vi "Read PL (2D) txt File.vi"(1 "Path":path) -> (0 "Intensity Graph":dbl[][](graph))   [LabVIEW 2011]
uses:
  <vilib>/Utility/file.llb/Read From Spreadsheet File (DBL).vi
panel:
  in  "Array":u32[](array[colorbox])
  in  "multiplier":dbl=13.79
  in  "start":dbl=13.79
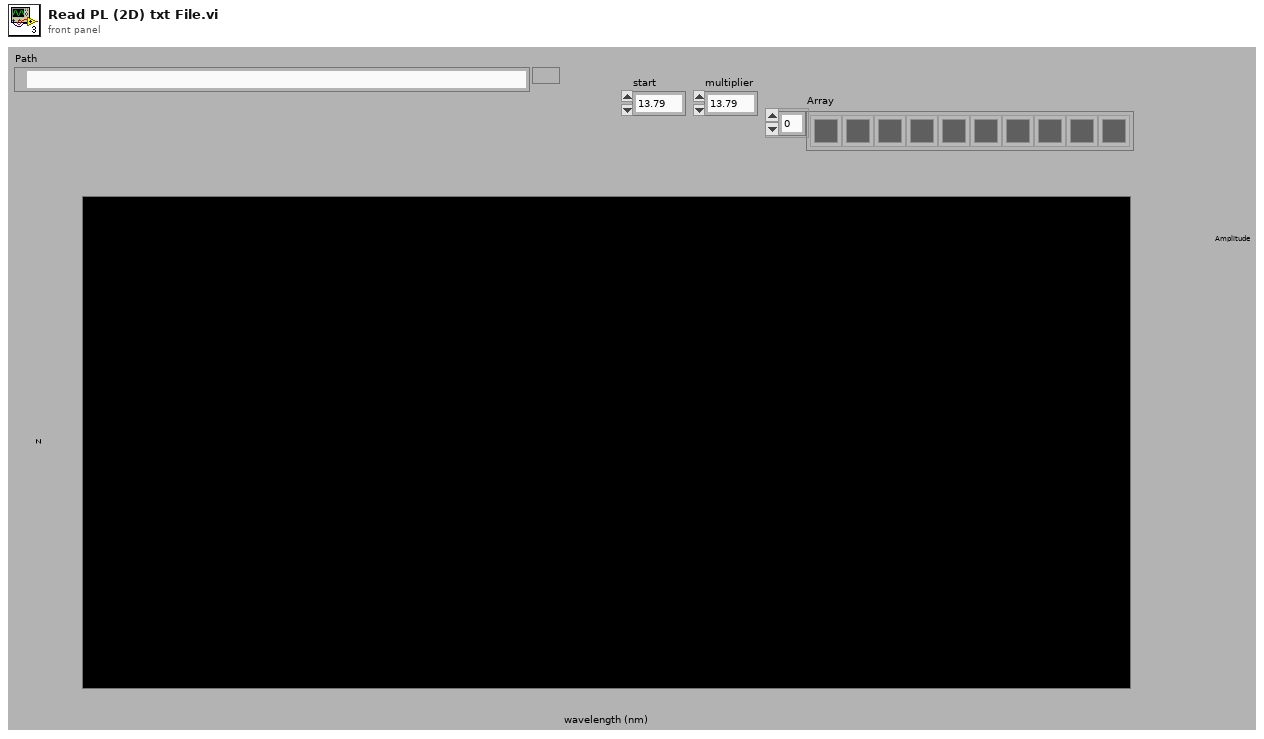
[diagram p1: front panel]
types:
  T1 = typedef "LVOffsetAndMultiplierTypeDef.ctl" = cluster{"Offset":dbl, "Multiplier":dbl}
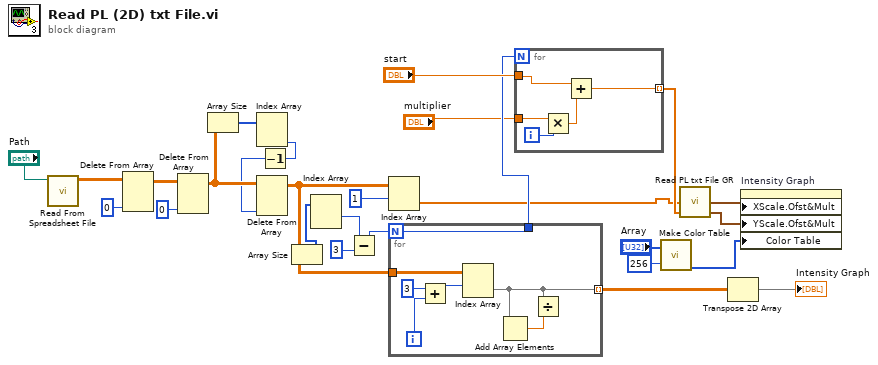
[diagram p0: block diagram]
diagram:
  n1 = call-poly <vilib>:"Read From Spreadsheet File.vi"("file path (dialog if empty)"="Path") -> ("all rows"=w24:dbl[][])  [unwired: 3 in, 7 out]
  n2 = Delete From Array(array=w24, index (col)=0 ("disabled index (col)")) -> (array with subset deleted=w27:dbl[][])  [unwired: 2 in, 1 out]
  n3 = Delete From Array(array=w27, index (col)=0 ("disabled index (col)")) -> (array with subset deleted=w22:dbl[][])  [unwired: 2 in, 1 out]
  n4 = Array Size(array=w22) -> (size(s)=w21:i32[])
  n5 = Index Array(array=w21) -> (element #2=w20:i32)  [unwired: 2 in, 1 out]
  n6 = Decrement(x=w20) -> (x-1=w19:i32)
  n7 = Delete From Array(array=w22, index (col)=w19) -> (array with subset deleted=w18:dbl[][])  [unwired: 2 in, 1 out]
  n8 = Array Size(array=w18) -> (size(s)=w17:i32[])
  n9 = Index Array(array=w17) -> (element #1=w14:i32)  [unwired: 2 in, 1 out]
  n10 = Subtract(x=w14, y=3 ("x")) -> (x-y=w15:i32)
  n11 = Index Array(array=w18, index (row)=1) -> (element=w6:dbl[])  [unwired: 1 in]
  n12 = for {
    N: w15 -> [w29]
    tunnel: w18 -> [w32]
    tunnel: [w28] -> w1 mode=indexing
    tunnel: [w29] -> w9
    i -> [w34]
    n13 = Add(x=3, y=w34) -> (x+y=w31:i32)
    n14 = Index Array(array=w32, index (row)=w31) -> (element=w28:dbl[])  [unwired: 1 in]
    n15 = Add Array Elements(numeric array=w28) -> (sum=w30:dbl)
    n16 = Divide(x=w28, y=w30) -> ()  [unwired: 1 out]
  }
  n17 = for {
    N: w9 -> [_]
    tunnel: "start" -> [w36]
    tunnel: "multiplier" -> [w38]
    tunnel: [w35] -> w7 mode=indexing
    i -> [w39]
    n18 = Multiply(x=w38, y=w39) -> (x*y=w37:dbl)
    n19 = Add(x=w36, y=w37) -> (x+y=w35:dbl)
  }
  n20 = call "Make Color Table.vi"("Array"="Array", "Size/3"=256) -> ("Color Tbl"=w5:u32[])  [unwired: 3 out]
  n21 = call "Read PL txt File GR.vi"("Y Scale"=w7, "X Scale"=w6) -> ("Y Scale.Offset and Multiplier"=w11:T1, "X Scale.Offset and Multiplier"=w13:T1)  [unwired: 1 in, 1 out]
  n22 = Transpose 2D Array(2D array=w1) -> (transposed array=→"Intensity Graph":dbl[][])
  n23 = property on="Intensity Graph" class="IntGraph (strict)"("XScale.Ofst&Mult"=w13, "YScale.Ofst&Mult"=w11, "Color Table"=w5) -> ()  [unwired: 2 in, 2 out]
